vi "emi_Get File name.vi"(0 "pre date string(\"\")":string, 1 "Time format(Data & Time)":T1(ring)=enum."Date & Time", 7 "post date string(\"\")":string, 9 "type name(\"dat\")":string="dat", 11 "error in (no error)":errorcluster) -> (8 "concatenated string":string, 15 "error out":errorcluster)   [LabVIEW 2011]
doc: "Create a file name based on inputs. Does not include path.\n\nPerformed regardless of error."
uses:
  Time/Private/emi_Time offset holder.vi
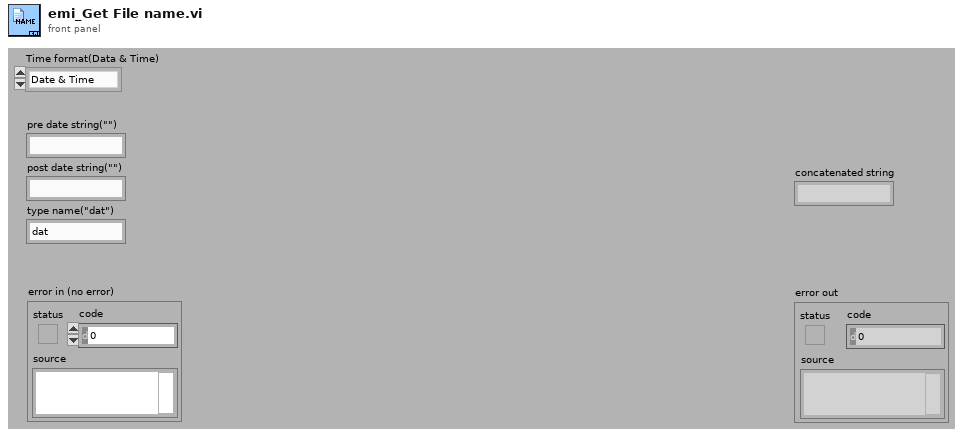
[diagram p1: front panel]
types:
  T1 = enum16{"Date & Time w ms", "Date & Time", "Time w ms", "Time", "Date", "Non"}
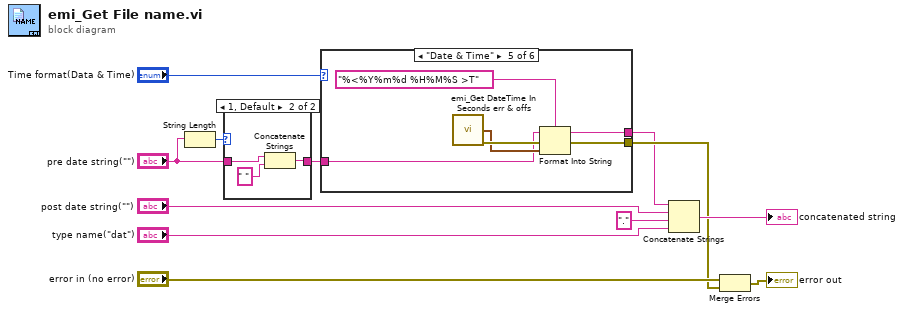
[diagram p0: block diagram]
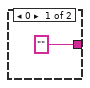
[diagram p2: hidden frame]
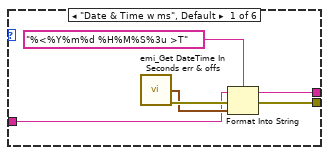
[diagram p3: hidden frame]
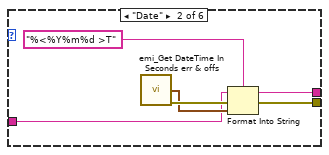
[diagram p4: hidden frame]
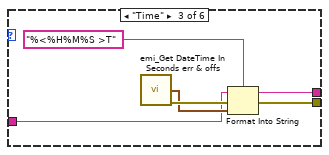
[diagram p5: hidden frame]
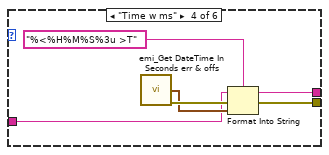
[diagram p6: hidden frame]
diagram:
  n1 = String Length(string="pre date string(\"\")") -> (length=w3:i32)
  n2 = case shown="1, Default" w3 {
    tunnel: ["" ("pre date string(\"\")") w16] -> w2
    tunnel: "pre date string(\"\")" -> [_ w15]
    frame 0 {
    }
    frame 1, Default {
      n3 = Concatenate Strings(w15, " " ("string")) -> (w16:string)
    }
  }
  n4 = case shown="\"Date & Time\"" "Time format(Data & Time)" {
    tunnel: [w20 w26 w32 w38 w44 _] -> w5
    tunnel: w2 -> [w19 w25 w31 w37 w43 w47]
    tunnel: [w17 w23 w29 w35 w41 w47] -> w4
    frame "Date & Time w ms", Default {
      n5 = call "emi_Get DateTime In Seconds err & offs.vi"() -> ("Time"=w21:timestamp, "error out"=w22:errorcluster)  [unwired: 14 in]
      n6 = Format Into String(format string="%<%Y%m%d %H%M%S%3u >T", initial string=w19, error in=w22, w21) -> (resulting string=w17:string, error out=w20:errorcluster)
    }
    frame "Date" {
      n7 = call "emi_Get DateTime In Seconds err & offs.vi"() -> ("Time"=w27:timestamp, "error out"=w28:errorcluster)  [unwired: 14 in]
      n8 = Format Into String(format string="%<%Y%m%d >T", initial string=w25, error in=w28, w27) -> (resulting string=w23:string, error out=w26:errorcluster)
    }
    frame "Time" {
      n9 = call "emi_Get DateTime In Seconds err & offs.vi"() -> ("Time"=w33:timestamp, "error out"=w34:errorcluster)  [unwired: 14 in]
      n10 = Format Into String(format string="%<%H%M%S >T", initial string=w31, error in=w34, w33) -> (resulting string=w29:string, error out=w32:errorcluster)
    }
    frame "Time w ms" {
      n11 = call "emi_Get DateTime In Seconds err & offs.vi"() -> ("Time"=w39:timestamp, "error out"=w40:errorcluster)  [unwired: 14 in]
      n12 = Format Into String(format string="%<%H%M%S%3u >T", initial string=w37, error in=w40, w39) -> (resulting string=w35:string, error out=w38:errorcluster)
    }
    frame "Date & Time" {
      n13 = call "emi_Get DateTime In Seconds err & offs.vi"() -> ("Time"=w45:timestamp, "error out"=w46:errorcluster)  [unwired: 14 in]
      n14 = Format Into String(format string="%<%Y%m%d %H%M%S >T", initial string=w43, error in=w46, w45) -> (resulting string=w41:string, error out=w44:errorcluster)
    }
    frame "Non" {
    }
  }
  n15 = Concatenate Strings(w4, "post date string(\"\")", "." ("string"), "type name(\"dat\")") -> (→"concatenated string":string)
  n16 = Merge Errors("error in (no error)", w5) -> (→"error out":errorcluster)
